vi "weideman64_dll.vi"() -> ()   [LabVIEW 2022 SP3]
panel:
  out "imag_out":dbl
  out "real_out":dbl
  in  "real_in":dbl
  in  "imag_in":dbl
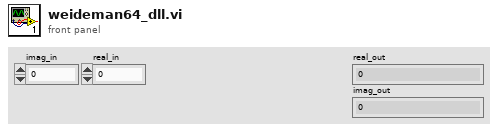
[diagram p1: front panel]
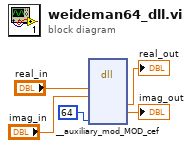
[diagram p0: block diagram]
diagram:
  n1 = dll-call lib="?" fn="__auxiliary_mod_MOD_cef"("arg1"="real_in", "arg2"="imag_in", "o"=64) -> ("arg3"=→"real_out":dbl, "i"=→"imag_out":dbl)  [unwired: 9 in, 2 out]
